vi "Wygladzanie.vi"(7 "Num (0..3)":i32, 11 "Array in":dbl[](array[numeric])) -> (3 "Array out":dbl[](array[numeric]))   [LabVIEW 2014]
panel:
  out "size(s) przetw":i32
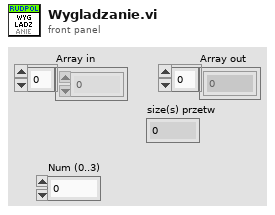
[diagram p1: front panel]
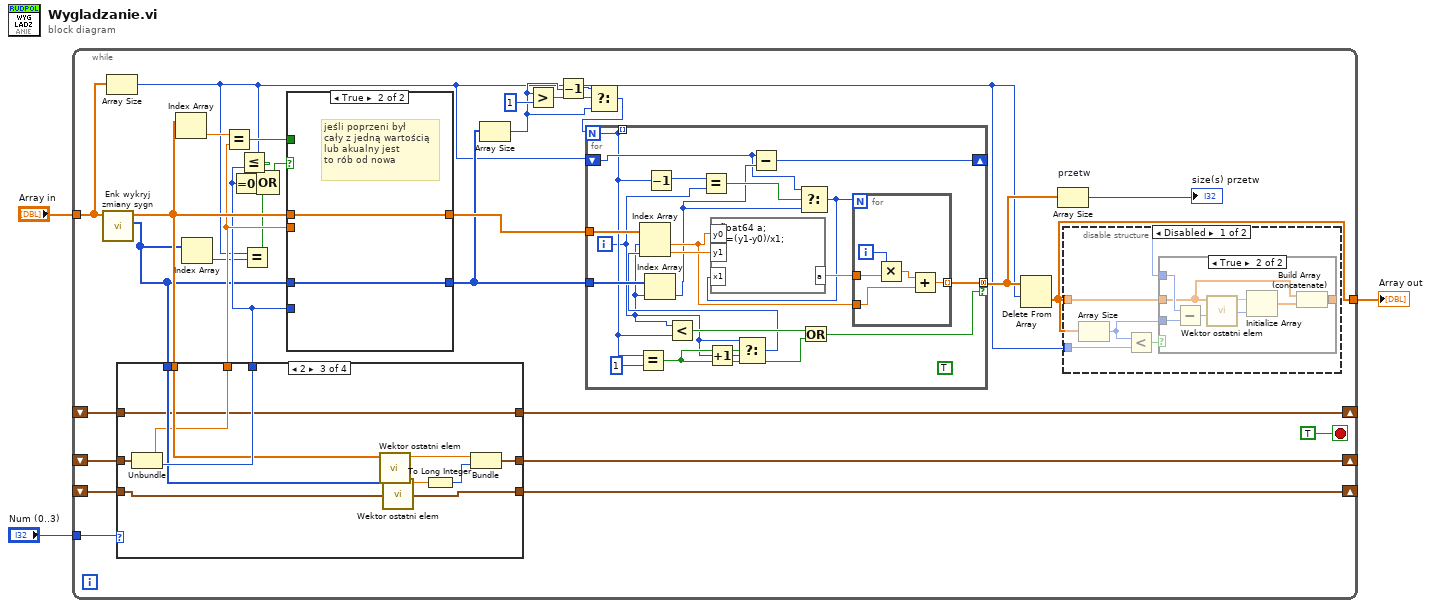
[diagram p0: block diagram]
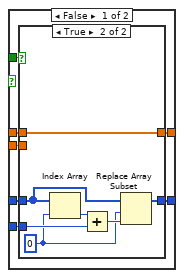
[diagram p2: hidden frame]
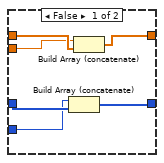
[diagram p3: hidden frame]
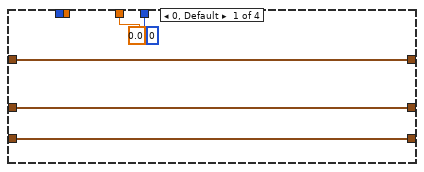
[diagram p6: hidden frame]
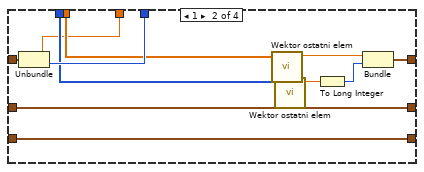
[diagram p7: hidden frame]
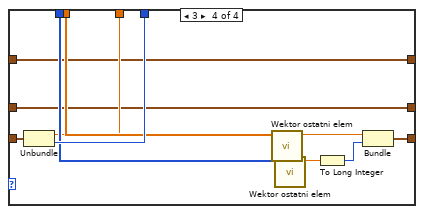
[diagram p8: hidden frame]
diagram:
  n1 = while {
    tunnel: "Array in" -> [w31]
    tunnel: [w24] -> w2
    shift-right: [w30] -> _
    shift-left: _ -> [w29]
    shift-right: [w21] -> _
    shift-left: _ -> [w18]
    shift-right: [w20] -> _
    shift-left: _ -> [w17]
    tunnel: "Num (0..3)" -> [w19]
    stop <- TRUE stop-if-true
    n2 = call "Enk wykryj zmiany sygn.vi"("Array in"=w31) -> ("l.probek"=w5:i32[], "skoki"=w27:dbl[])  [unwired: 9 in]
    n3 = Array Size(array=w31) -> (size(s)=w6:i32)
    n4 = case shown="2" w19 {
      tunnel: [w73 w76 w87 w98] -> w30
      tunnel: w29 -> [w73 w84 w87 w98]
      tunnel: [0 w83 w95 w106] -> w11
      tunnel: w27 -> [_ w82 w94 w105]
      tunnel: w5 -> [_ w80 w92 w103]
      tunnel: [0.0 ("ostatni") w77 w89 w100] -> w25
      tunnel: [w72 w75 w85 w96] -> w21
      tunnel: [w71 w74 w86 w99] -> w20
      tunnel: w18 -> [w72 w75 w88 w96]
      tunnel: w17 -> [w71 w74 w86 w97]
      frame 0, Default {
      }
      frame 1 {
        n5 = Unbundle(w84) -> ("ostatni"=w77:dbl, w83:i32)
        n6 = call "Wektor ostatni elem.vi"("wektor"=w82) -> ("ostatni"=w81:dbl)  [unwired: 10 in]
        n7 = call "Wektor ostatni elem.vi"("wektor"=w80) -> ("ostatni"=w79:dbl)  [unwired: 10 in]
        n8 = To Long Integer(number=w79) -> (32bit integer=w78:i32)
        n9 = Bundle("ostatni"=w81, w78) -> (w76:cluster{"ostatni":dbl, i32})  [unwired: 1 in]
      }
      frame 2 {
        n10 = Unbundle(w88) -> ("ostatni"=w89:dbl, w95:i32)
        n11 = call "Wektor ostatni elem.vi"("wektor"=w94) -> ("ostatni"=w93:dbl)  [unwired: 10 in]
        n12 = call "Wektor ostatni elem.vi"("wektor"=w92) -> ("ostatni"=w91:dbl)  [unwired: 10 in]
        n13 = To Long Integer(number=w91) -> (32bit integer=w90:i32)
        n14 = Bundle("ostatni"=w93, w90) -> (w85:cluster{"ostatni":dbl, i32})  [unwired: 1 in]
      }
      frame 3 {
        n15 = Unbundle(w97) -> ("ostatni"=w100:dbl, w106:i32)
        n16 = call "Wektor ostatni elem.vi"("wektor"=w105) -> ("ostatni"=w104:dbl)  [unwired: 10 in]
        n17 = call "Wektor ostatni elem.vi"("wektor"=w103) -> ("ostatni"=w102:dbl)  [unwired: 10 in]
        n18 = To Long Integer(number=w102) -> (32bit integer=w101:i32)
        n19 = Bundle("ostatni"=w104, w101) -> (w99:cluster{"ostatni":dbl, i32})  [unwired: 1 in]
      }
    }
    n20 = Index Array(array=w27) -> (element=w34:dbl)  [unwired: 1 in]
    n21 = Index Array(array=w5) -> (element=w4:i32)  [unwired: 1 in]
    n22 = Equal?(x=w34, y=w25) -> (x = y?=w33:bool)
    n23 = Equal To 0?(x=w11) -> (x = 0?=w8:bool)
    n24 = Less Or Equal?(x=w6, y=w11) -> (x <= y?=w9:bool)
    n25 = Equal?(x=w6, y=w4) -> (x = y?=w7:bool)
    n26 = Compound Arithmetic op=OR(w9, w8, w7) -> (w10:bool)
    n27 = case shown="True" w10 {
      tunnel: w33 -> [w41 _]
      tunnel: [w40 w56] -> w28
      tunnel: w27 -> [w39 w56]
      tunnel: w5 -> [w38 w55]
      tunnel: [w37 w55] -> w26
      tunnel: w25 -> [w36 _]
      tunnel: w11 -> [w35 _]
      frame False {
        n28 = case shown="True" w41 {
          tunnel: w39 -> [w47 w52]
          tunnel: [w46 w52] -> w40
          tunnel: w38 -> [w44 w51]
          tunnel: [w43 w49] -> w37
          tunnel: w35 -> [w42 w53]
          tunnel: w36 -> [w45 _]
          frame False {
            n29 = Build Array (concatenate)(w42, w44) -> (w43:i32[])
            n30 = Build Array (concatenate)(w45, w47) -> (w46:dbl[])
          }
          frame True {
            w48 = 0 ("index")
            n31 = Index Array(array=w51, index=w48) -> (element=w54:i32)
            n32 = Add(x=w54, y=w53) -> (x+y=w50:i32)
            n33 = Replace Array Subset(array=w51, new element=w50, index=w48) -> (w49:i32[])
          }
        }
      }
      frame True {
        # "jeśli poprzeni był\ncały z jedną wartością\nlub akualny jest\nto rób od nowa"
      }
    }
    n34 = Array Size(array=w26) -> (size(s)=w12:i32)
    n35 = Greater?(x=w12, y=1) -> (0:w15:bool)
    n36 = Decrement(x=w12) -> (x-1=w13:i32)
    n37 = Select(t=w13, s=w15, f=w12) -> (s? t:f=w14:i32)
    n38 = for {
      N: w14 -> [w112]
      tunnel: w28 -> [w126]
      tunnel: [w122] -> w23 mode=concatenating if=w114
      tunnel: w26 -> [w120]
      shift-right: [w117] -> _
      shift-left: w6 -> [w115]
      tunnel: [w112] -> _ mode=indexing
      i -> [w107]
      (unwired) TRUE
      n39 = Equal?(x=w112, y=1) -> (x = y?=w110:bool)
      n40 = Index Array(array=w120, index=w107) -> (element=w116:i32)
      n41 = Decrement(x=w112) -> (x-1=w119:i32)
      n42 = Less?(x=w107, y=w112) -> (x < y?=w111:bool)
      n43 = Equal?(x=w119, y=w107) -> (x = y?=w118:bool)
      n44 = Increment(x=w107) -> (x+1=w108:i32)
      n45 = Select(t=w107, s=w110, f=w108) -> (s? t:f=w109:i32)
      n46 = Index Array(array=w126, index #1=w107, index #2=w109) -> (element #1=w123:dbl, element #2=w125:dbl)
      n47 = Subtract(x=w115, y=w116) -> (x-y=w117:i32)
      n48 = Select(t=w115, s=w118, f=w116) -> (s? t:f=w113:i32)
      n49 = formula code="float64 a;\na=(y1-y0)/x1;"("y0"=w123, "y1"=w125, "x1"=w113) -> ("a"=w124:dbl)
      n50 = Or(x=w111, y=w110) -> (x .or. y?=w114:bool)
      n51 = for {
        N: w113 -> [_]
        tunnel: w124 -> [w131]
        tunnel: w123 -> [w128]
        tunnel: [w127] -> w122 mode=indexing
        i -> [w130]
        n52 = Multiply(x=w130, y=w131) -> (x*y=w129:dbl)
        n53 = Add(x=w129, y=w128) -> (x+y=w127:dbl)
      }
    }
    n54 = Delete From Array(array=w23, length=w6) -> (deleted portion=w24:dbl[])  [unwired: 1 in, 1 out]
    n55 = Array Size "przetw"(array=w23) -> (size(s)=→"size(s) przetw":i32)
    n56 = disable-structure shown="Disabled" {
      disable-tunnel: w24 -> [w58 _]
      disable-tunnel: w6 -> [w57 _]
      frame Disabled {
        n57 = Array Size(array=w58) -> (size(s)=w59:i32)
        n58 = Less?(x=w59, y=w57) -> (x < y?=w60:bool)
        n59 = case shown="True" w60 {
          tunnel: w58 -> [w61 w63]
          tunnel: [w61 w62] -> _
          tunnel: w57 -> [_ w68]
          tunnel: w59 -> [_ w67]
          frame False {
          }
          frame True {
            n60 = Subtract(x=w68, y=w67) -> (x-y=w65:i32)
            n61 = call "Wektor ostatni elem.vi"("wektor"=w63) -> ("ostatni"=w66:dbl)  [unwired: 10 in]
            n62 = Initialize Array(w66, w65) -> (w64:dbl[])
            n63 = Build Array (concatenate)(w63, w64) -> (w62:dbl[])
          }
        }
      }
      frame Enabled {
      }
    }
  }
  "Array out" <- w2
